vi "Check For Full Board.vi"(8 "error in (no error)":errorcluster, 11 "Game Engine in":refnum<class "Game Engine.lvclass">) -> (0 "error out":errorcluster, 2 "Pieces are Out of Bounds":bool, 3 "Game Engine out":refnum<class "Game Engine.lvclass">)   [LabVIEW 2017, in "Game Engine.lvlib" / "Game Engine.lvclass"]
uses:
  Game Engine.lvclass
  Game Engine.lvclass/Game Engine.ctl
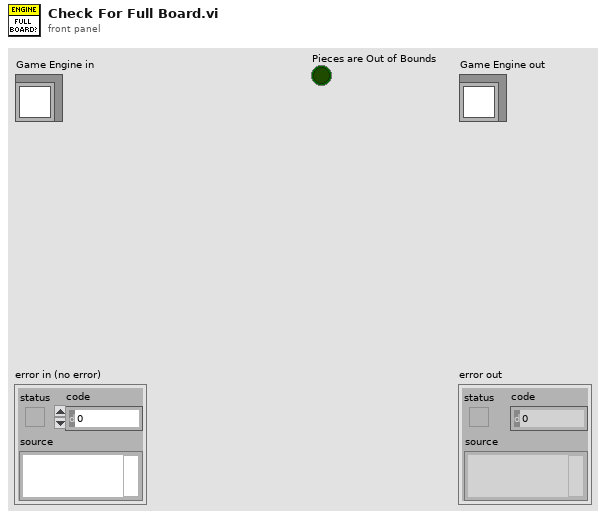
[diagram p1: front panel]
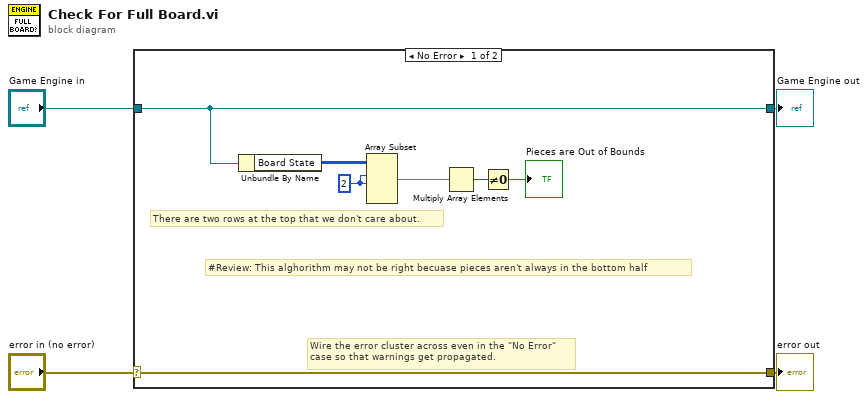
[diagram p0: block diagram]
diagram:
  n1 = case shown="No Error" "error in (no error)" {
    selector: "error in (no error)" -> [w11 w13]
    tunnel: [w11 w13] -> w3
    tunnel: [w10 w12] -> w1
    tunnel: "Game Engine in" -> [w10 w12]
    frame No Error {
      w5 = 2 ("length")
      # "There are two rows at the top that we don't care about."
      # "#Review: This alghorithm may not be right becuase pieces aren't always in the bottom half"
      # "Wire the error cluster across even in the \"No Error\"\ncase so that warnings get propagated."
      n2 = Unbundle By Name(w10) -> ("Board State"=w9:u32[][])
      n3 = Array Subset(array=w9, index (row)=w5, length (row)=w5) -> (w8:u32[][])  [unwired: 2 in]
      n4 = Multiply Array Elements(1:w8) -> (0:w7:u32)
      n5 = Not Equal To 0?(x=w7) -> (x != 0?=→"Pieces are Out of Bounds":bool)
    }
    frame Error {
    }
  }
  "error out" <- w3
  "Game Engine out" <- w1
